vi "Example.vi"() -> ()   [LabVIEW 2009]
uses:
  CRC SubVIs/Inline CRC-32.vi
  CRC SubVIs/Wrappers/CRC-16-CCITT-0x1D0F.vi
  CRC SubVIs/Wrappers/CRC-16-CCITT-0xFFFF.vi
  CRC SubVIs/Wrappers/CRC-16-CCITT-xMODEM.vi
  CRC SubVIs/Wrappers/CRC-8-CCITT.vi
  CRC SubVIs/Wrappers/CRC-8-Maxim 1-Wire (DOW).vi
panel:
  out "CRC-8-Maxim 1-Wire (DOW)":u8 format="%.0x"
  out "CRC-8-CCITT":u8 format="%.0x"
  out "CRC-16-CCITT-xModem":u16 format="%.0x"
  out "CRC-16-CCITT-0xFFFF":u16 format="%.0x"
  out "CRC-16-CCITT-0x1D0F":u16 format="%.0x"
  out "CRC-32":u32 format="%.0x"
  in  "String":string="this is a test string"
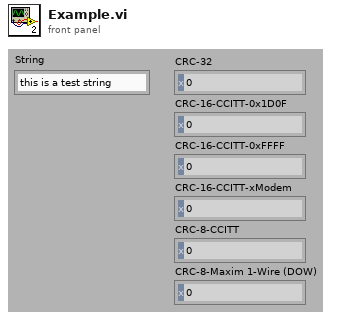
[diagram p1: front panel]
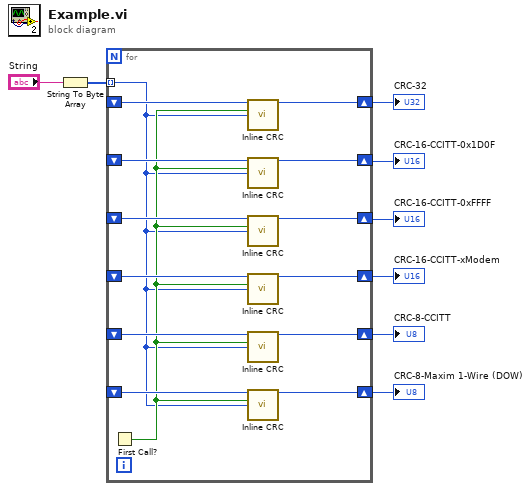
[diagram p0: block diagram]
diagram:
  n1 = String To Byte Array(string="String") -> (unsigned byte array=w7:u8[])
  n2 = for {
    shift-right: [w22] -> w6
    shift-left: _ -> [w21]
    shift-right: [w20] -> w5
    shift-left: _ -> [w15]
    shift-right: [w19] -> w4
    shift-left: _ -> [w14]
    shift-right: [w18] -> w3
    shift-left: _ -> [w13]
    shift-right: [w17] -> w2
    shift-left: _ -> [w12]
    shift-right: [w16] -> w1
    shift-left: _ -> [w11]
    tunnel: w7 -> [w9] mode=indexing
    n3 = First Call?() -> (First Call?: T/F=w10:bool)
    n4 = call-poly "Inline CRC.vi"("CRC In"=w21, "Reset"=w10, "Data"=w9) -> ("CRC"=w22:u32)  [unwired: 11 in, 1 out]
    n5 = call-poly "Inline CRC.vi"("CRC In"=w15, "Reset"=w10, "Data"=w9) -> ("CRC"=w20:u16)  [unwired: 11 in, 1 out]
    n6 = call-poly "Inline CRC.vi"("CRC In"=w14, "Reset"=w10, "Data"=w9) -> ("CRC"=w19:u16)  [unwired: 11 in, 1 out]
    n7 = call-poly "Inline CRC.vi"("CRC In"=w13, "Reset"=w10, "Data"=w9) -> ("CRC"=w18:u16)  [unwired: 11 in, 1 out]
    n8 = call-poly "Inline CRC.vi"("CRC In"=w12, "Reset"=w10, "Data"=w9) -> ("CRC"=w17:u8)  [unwired: 11 in, 1 out]
    n9 = call-poly "Inline CRC.vi"("CRC In"=w11, "Reset"=w10, "Data"=w9) -> ("CRC"=w16:u8)  [unwired: 11 in, 1 out]
  }
  "CRC-32" <- w6
  "CRC-16-CCITT-0x1D0F" <- w5
  "CRC-16-CCITT-0xFFFF" <- w4
  "CRC-16-CCITT-xModem" <- w3
  "CRC-8-CCITT" <- w2
  "CRC-8-Maxim 1-Wire (DOW)" <- w1
